vi "DllFxpAddSub_Bool.vi"(6 "cin/nbin":bool, 8 "load":bool=TRUE, 9 "is sub":bool, 10 "y":bool, 11 "x":bool) -> (2 "cout/nbout/overflow":bool, 3 "s":bool)   [LabVIEW 2017]
uses:
  <vilib>/rvi/FXPMathLib/sim/FxpSim.dll
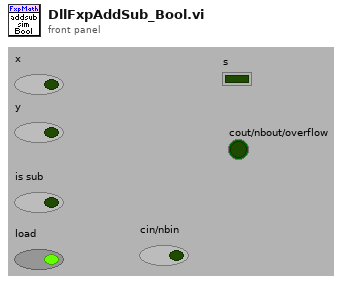
[diagram p1: front panel]
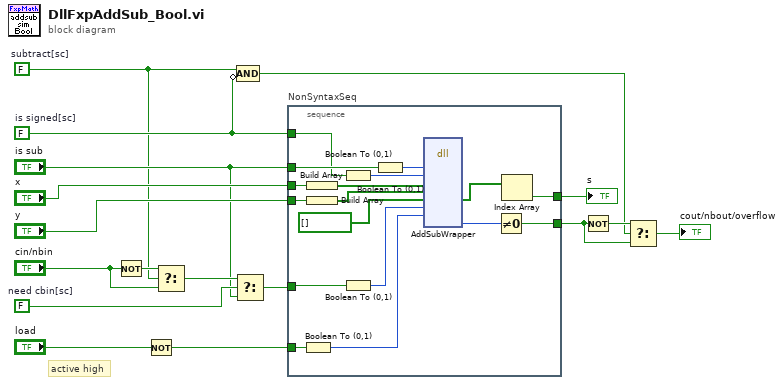
[diagram p0: block diagram]
diagram:
  w2 = FALSE  # subtract[sc]
  w3 = FALSE  # is signed[sc]
  w17 = FALSE  # need cbin[sc]
  # "active high"
  n1 = Not(x="cin/nbin") -> (.not. x?=w8:bool)
  n2 = Not(x="load") -> (.not. x?=w10:bool)
  n3 = Select(t=w8, s=w2, f="cin/nbin") -> (s? t:f=w11:bool)
  n4 = Select(t=w11, s=w17, f="is sub") -> (s? t:f=w16:bool)
  n5 = Compound Arithmetic op=AND(w2, invert w3) -> (w1:bool)
  n6 = stacked-sequence "NonSyntaxSeq" {
    tunnel: [w34] -> w5
    tunnel: "is sub" -> [w33]
    tunnel: w16 -> [w30]
    tunnel: w10 -> [w29]
    tunnel: w3 -> [w28]
    tunnel: [w27] -> w14
    tunnel: "x" -> [w26]
    tunnel: "y" -> [w23]
    frame #0 {
      n7 = Boolean To (0,1)(Boolean=w29) -> (0, 1=w21:i16)
      n8 = Build Array(w26) -> (w25:bool[])
      n9 = Build Array(w23) -> (w24:bool[])
      n10 = Boolean To (0,1)(Boolean=w28) -> (0, 1=w31:i16)
      n11 = Boolean To (0,1)(Boolean=w30) -> (0, 1=w20:i16)
      n12 = Boolean To (0,1)(Boolean=w33) -> (0, 1=w32:i16)
      n13 = dll-call lib="e:/penguin/lvdist/win32/export/17.0/17.0.1f1/dist/vi.lib/rvi/FXPMathLib/sim/FxpSim.dll" fn="AddSubWrapper"("isSub"=w32, "isSigned"=w31, "xH"=w25, "yH"=w24, "zH"=bool[] [] ("xH"), "CinOrNBin"=w20, "notLoad"=w21) -> ("zH"=w18:bool[], "CoutOrNBoutOrOvfl"=w22:u8)  [unwired: 5 in, 8 out]
      n14 = Not Equal To 0?(x=w22) -> (x != 0?=w34:bool)
      n15 = Index Array(array=w18) -> (element=w27:bool)  [unwired: 1 in]
    }
  }
  "s" <- w14
  n16 = Not(x=w5) -> (.not. x?=w6:bool)
  n17 = Select(t=w6, s=w1, f=w5) -> (s? t:f=→"cout/nbout/overflow":bool)
